vi "TimeSeriesChart.vi"(6 "IncomingLength":i32=820, 7 "String":string, 8 "iStep":i32=819, 9 "errors":bool[](array[boolean])=[FALSE, FALSE, FALSE, FALSE, FALSE], 10 "VmagUVWCone":dbl[](array[numeric])=[4.652117426792975, 3.8906570585724807, -2.52811200323062, -0.33709628353377885, 33.24650333523261] caption="Vmag                      U                        V                           W                      Cone", 11 "netPressures":dbl[](array[numeric])=[3.067774207341401, 2.2293825655100505, 2.8603385138725983, 3.5535614729171847, 1.9395849612811382]) -> ()   [LabVIEW 2013]
uses:
  5HPGraph.ctl
  <vilib>/Waveform/DWDTOps.llb/DWDT Analog to Digital.vi
panel:
  out "5HP diagnostic graph":T1
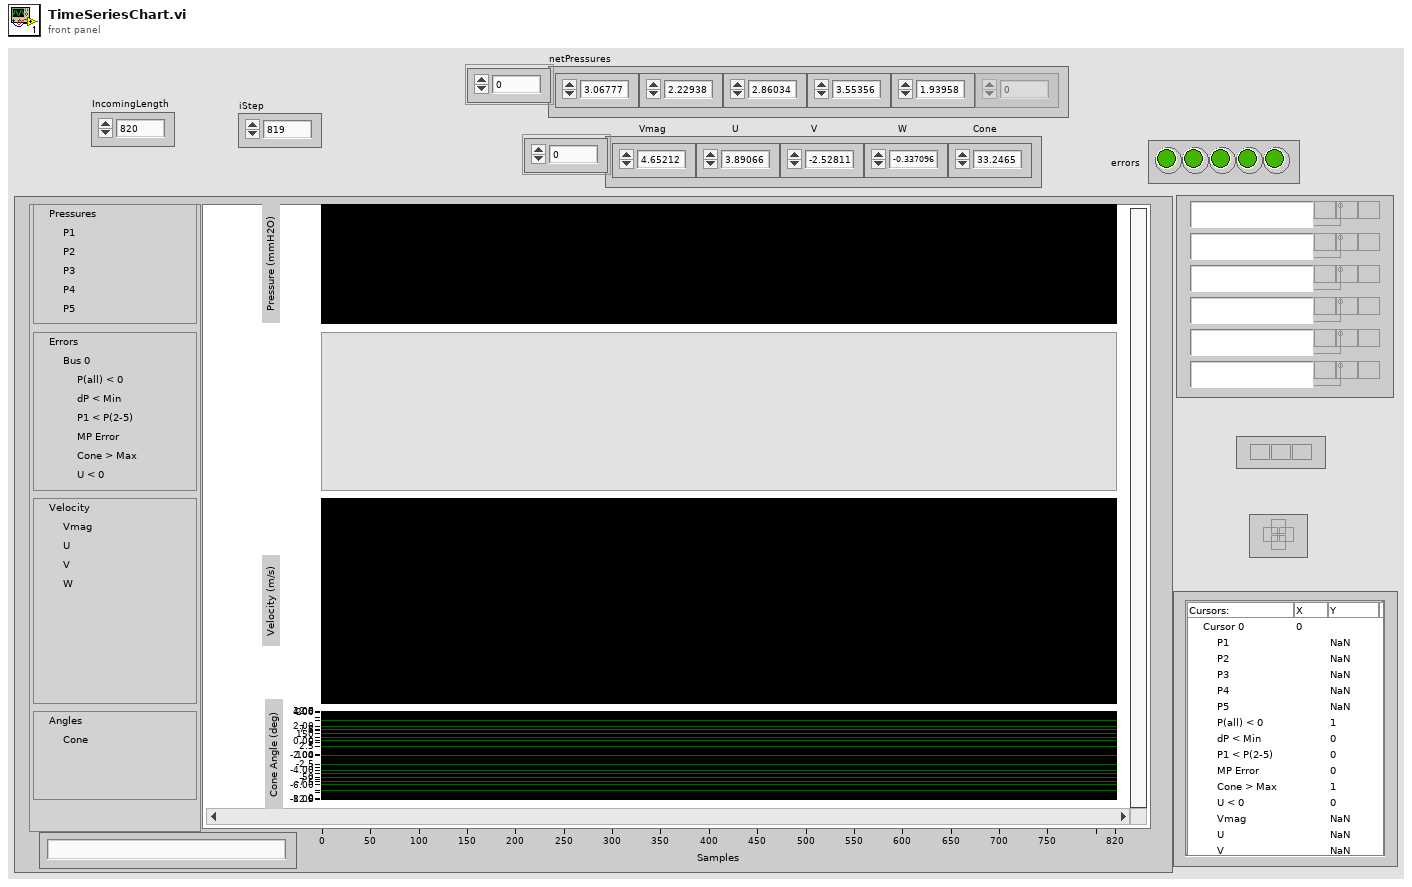
[diagram p1: front panel]
types:
  T1 = typedef "5HPGraph.ctl" = cluster{dbl[][], "digital waveform":digitalwaveform, dbl[][]}
  T2 = cluster{string, u32, enum16{"Pressures", "Errors", "Velocity", "Angles"}}[]
  T3 = enum16{"Pressures", "Errors", "Velocity", "Angles"}
  T4 = cluster{dbl[][], "digital waveform":digitalwaveform, dbl[][]}
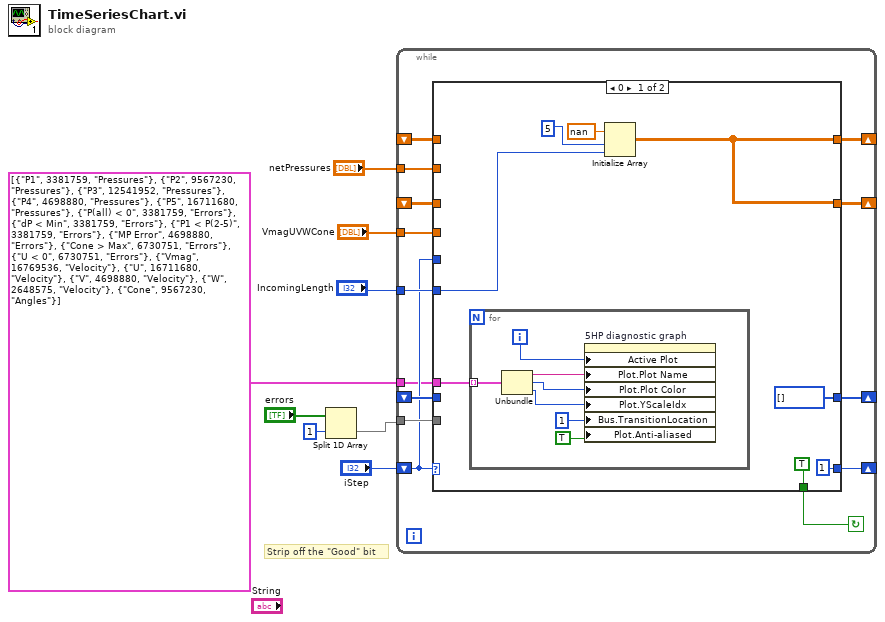
[diagram p0: block diagram]
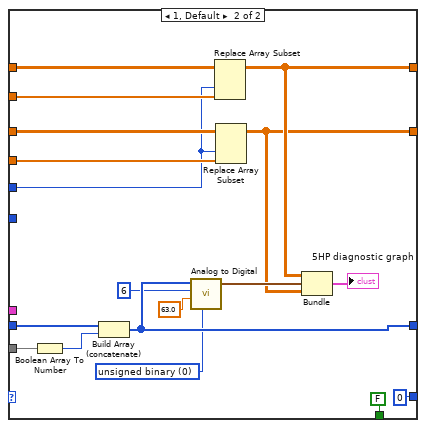
[diagram p2: hidden frame]
diagram:
  # "Strip off the \"Good\" bit"
  n1 = Split 1D Array(array="errors", index=1) -> (second subarray=w2:bool[])  [unwired: 1 out]
  n2 = while {
    shift-right: [w19] -> _
    shift-left: _ -> [w20]
    tunnel: "netPressures" -> [w22]
    tunnel: "VmagUVWCone" -> [w21]
    shift-right: [w17] -> _
    shift-left: "iStep" -> [w12]
    tunnel: w2 -> [w16]
    shift-right: [w14] -> _
    shift-left: _ -> [w15]
    tunnel: "IncomingLength" -> [w13]
    shift-right: [w10] -> _
    shift-left: _ -> [w11]
    tunnel: T2 [{"P1", 3381759, enum."Pressures"}, {"P2", 9567230, enum."Pressures"}, {"P3", 12541952, enum."Pressures"}, {"P4", 4698880, enum."Pressures"}, {"P5", 16711680, enum."Pressures"}, {"P(all) < 0", 3381759, enum."Errors"}, {"dP < Min", 3381759, enum."Errors"}, {"P1 < P(2-5)", 3381759, enum."Errors"}, {"MP Error", 4698880, enum."Errors"}, {"Cone > Max", 6730751, enum."Errors"}, {"U < 0", 6730751, enum."Errors"}, {"Vmag", 16769536, enum."Velocity"}, {"U", 16711680, enum."Velocity"}, {"V", 4698880, enum."Velocity"}, {"W", 2648575, enum."Velocity"}, {"Cone", 9567230, enum."Angles"}] -> [w9]
    stop <- w18 continue-if-true
    n3 = case shown="0" w12 {
      tunnel: w22 -> [_ w43]
      tunnel: w21 -> [_ w41]
      tunnel: w20 -> [_ w45]
      tunnel: [w24 w39] -> w19
      tunnel: [TRUE FALSE] -> w18
      tunnel: [1 0] -> w17
      tunnel: w16 -> [_ w53]
      tunnel: w15 -> [_ w51]
      tunnel: [u32[] [] w50] -> w14
      tunnel: w13 -> [w25 _]
      tunnel: w12 -> [_ w40]
      tunnel: w11 -> [_ w42]
      tunnel: [w24 w38] -> w10
      tunnel: w9 -> [w23 _]
      frame 0 {
        n4 = for {
          tunnel: w23 -> [w36] mode=indexing
          i -> [w37]
          n5 = Unbundle(w36) -> (w35:string, w34:u32, w33:T3)
          n6 = property on="5HP diagnostic graph" class="MixedGraph (strict)"("Active Plot"=w37, "Plot.Plot Name"=w35, "Plot.Plot Color"=w34, "Plot.YScaleIdx"=w33, "Bus.TransitionLocation"=u8 1 ("Bus.Digital Transition Location"), "Plot.Anti-aliased"=TRUE) -> ()  [unwired: 2 in, 2 out]
        }
        n7 = Initialize Array(nan ("element"), 5 ("dimension size"), w25) -> (w24:dbl[][])
      }
      frame 1, Default {
        w47 = u16 0 items=["unsigned binary", "offset binary", "2's complement"] ("data format (offset binary)")
        n8 = Boolean Array To Number(Boolean array=w53) -> (number=w52:u32)
        n9 = Build Array (concatenate)(w51, w52) -> (w50:u32[])
        n10 = call-poly <vilib>:"Analog to Digital.vi"("data format (offset binary)"=w47, "full-scale range (pk-pk)"=63.0, "resolution (16 bit)"=6, "analog waveform"=w50) -> ("digital waveform"=w49:digitalwaveform)  [unwired: 4 in, 3 out]
        n11 = Replace Array Subset(array=w45, new element=w43, index (col)=w40) -> (w39:dbl[][])  [unwired: 1 in]
        n12 = Replace Array Subset(array=w42, new element=w41, index (col)=w40) -> (w38:dbl[][])  [unwired: 1 in]
        n13 = Bundle(w39, "digital waveform"=w49, w38) -> (→"5HP diagnostic graph":T4)  [unwired: 1 in]
      }
    }
  }
